vi "Error Query.vi"(8 "error in (no error)":errorcluster, 11 "VISA resource name":refnum<visa-resource-name>) -> (0 "error out":errorcluster, 1 "Error Message":string, 2 "Error Code":i32[](array[numeric]), 3 "VISA resource name out":refnum<visa-resource-name>)   [LabVIEW 2023, in "Agilent ENA Series.lvlib"]
doc: "Queries the instrument for any errors in the instrument's error queue. It will continue to read errors until all errors have been read from the instrument. Any errors will be returned in the Error Out cluster.\n\nNote:\nThis VI is called automatically by most driver VIs so it is not usually necessary to call this in an application."
uses:
  Agilent ENA Series.lvlib
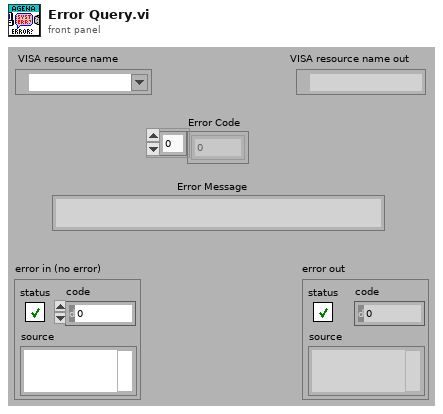
[diagram p1: front panel]
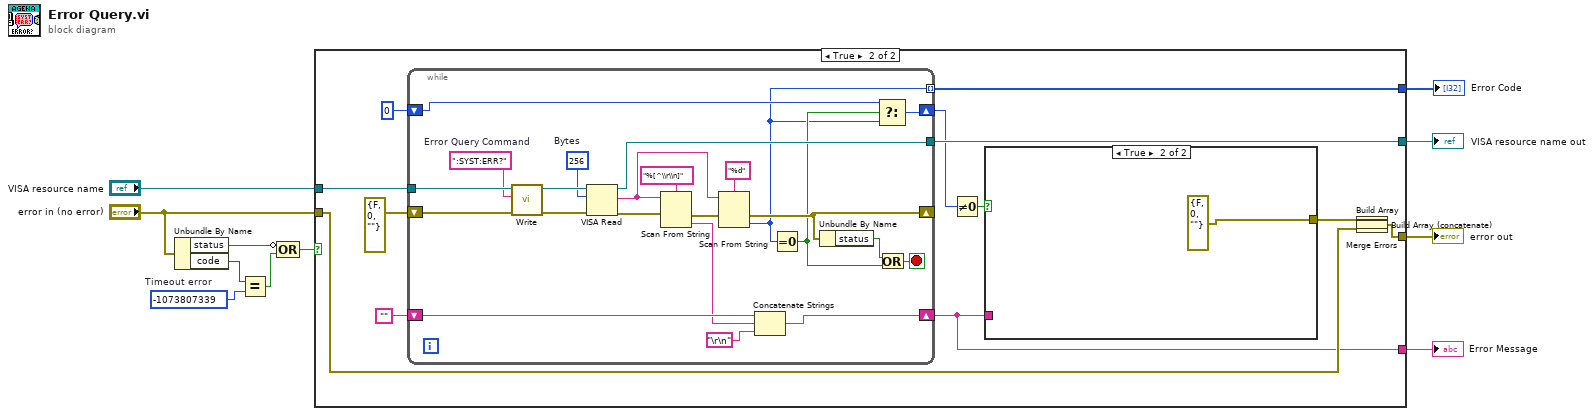
[diagram p0: block diagram]
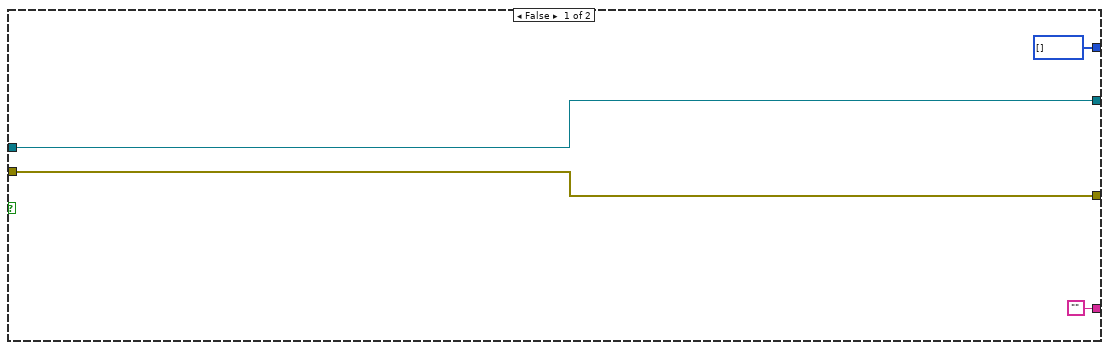
[diagram p2: hidden frame]
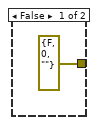
[diagram p3: hidden frame]
diagram:
  w6 = -1073807339  # Timeout error
  n1 = Unbundle By Name("error in (no error)") -> ("status"=w7:bool, "code"=w4:i32)
  n2 = Equal?(x=w4, y=w6) -> (x = y?=w5:bool)
  n3 = Compound Arithmetic op=OR(invert w7, w5) -> (w3:bool)
  n4 = case shown="True" w3 {
    tunnel: [w15 w29] -> w11
    tunnel: "VISA resource name" -> [w15 w28]
    tunnel: "error in (no error)" -> [w14 w22]
    tunnel: [w14 w26] -> w9
    tunnel: ["" w19] -> w2
    tunnel: [i32[] [] w18] -> w1
    frame False {
    }
    frame True {
      n5 = while {
        tunnel: [w54] -> w29
        tunnel: w28 -> [w53]
        shift-right: [w41] -> w19
        shift-left: "" -> [w44]
        shift-right: [w39] -> w20
        shift-left: 0 -> [w40]
        shift-right: [w37] -> _
        shift-left: errorcluster {"status"=FALSE, "code"=0, "source"=""} ("error in (no error)") -> [w38]
        tunnel: [w32] -> w18 mode=indexing
        stop <- w47 stop-if-true
        w51 = u32 256  # Bytes
        w49 = ":SYST:ERR?"  # Error Query Command
        n6 = call "Write.vi"("error in (no error)"=w38, "String ()"=w49, "VISA resource name"=w53) -> ("error out"=w50:errorcluster, "VISA resource name out"=w52:refnum<visa-resource-name>)  [unwired: 6 in, 1 out]
        n7 = VISA Read(VISA resource name=w52, byte count=w51, error in (no error)=w50) -> (VISA resource name out=w54:refnum<visa-resource-name>, read buffer=w45:string, error out=w36:errorcluster)  [unwired: 1 out]
        n8 = Scan From String(format string="%[^\\r\\n]", input string=w45, error in=w36) -> (error out=w35:errorcluster, output 1=w42:string)  [unwired: 2 in, 2 out]
        n9 = Scan From String(format string="%d", input string=w45, error in=w35) -> (error out=w37:errorcluster, output 1=w32:i32)  [unwired: 2 in, 2 out]
        n10 = Concatenate Strings(w44, w42, "\r\n") -> (w41:string)
        n11 = Equal To 0?(x=w32) -> (x = 0?=w33:bool)
        n12 = Unbundle By Name(w37) -> ("status"=w34:bool)
        n13 = Select(t=w40, s=w33, f=w32) -> (s? t:f=w39:i32)
        n14 = Or(x=w34, y=w33) -> (x .or. y?=w47:bool)
      }
      n15 = Not Equal To 0?(x=w20) -> (x != 0?=w24:bool)
      n16 = case shown="True" w24 {
        tunnel: w19 -> [_ _]
        tunnel: [errorcluster {"status"=FALSE, "code"=0, "source"=""} ("error out") errorcluster {"status"=FALSE, "code"=0, "source"=""} ("error out")] -> w23
        frame False {
        }
        frame True {
        }
      }
      n17 = Build Array(w23, w22) -> (w17:errorcluster[])
      n18 = Build Array (concatenate)(w17) -> (w16:errorcluster[])
      n19 = Merge Errors(w16) -> (w26:errorcluster)
    }
  }
  "VISA resource name out" <- w11
  "error out" <- w9
  "Error Message" <- w2
  "Error Code" <- w1
